vi "evaluation.vi"() -> ()   [LabVIEW 2017]
panel:
  in  "行程测试":bool
  in  "控制板调试":bool
  out "周期稳定性":dbl[](array[numeric])
  out "线性传感器基本误差":dbl[](array[numeric])
  out "重复性误差 R":dbl[](array[numeric])
  out "线性误差":dbl[](array[numeric])
  out "压力传感器系统误差 LH":dbl[](array[numeric])
  out "满量程输出yfs V":dbl[](array[numeric])
  out "温漂":dbl[](array[numeric])
  out "迟滞":dbl[](array[numeric])
  in  "计算参数":bool
  in  "退出":bool
  out "常温索引":i32
  out "XY图":cluster{dbl[], dbl[]}(graph)
  out "显示曲线界面":cluster{dbl[], dbl[]}[][](array[cluster])
  in  "传感器曲线图显示":T1(ring)
  in  "压力下限kPa":dbl
  in  "压力上限kPa":dbl=15000.0
  out "时漂":dbl[](array[numeric])
  out "曲线信息":string[][](array[string])
  in  "压力点个数":i32=6
  in  "检定次数":i32=3
  in  "行程采集文件名":string="202293_1902_700"
  in  "时漂文件名":string="2022917_1702_20.0"
  # "多通道 传感器评估系统"
  # "1"
  # "2"
  # "3"
  # "4"
  # "5"
  # "6"
  # "7"
  # "8"
  # "9"
  # "10"
  # "注意：\n请在计算参数前，先进行行程测试。\n选择传感器索引，获取相关传感器曲线图。"
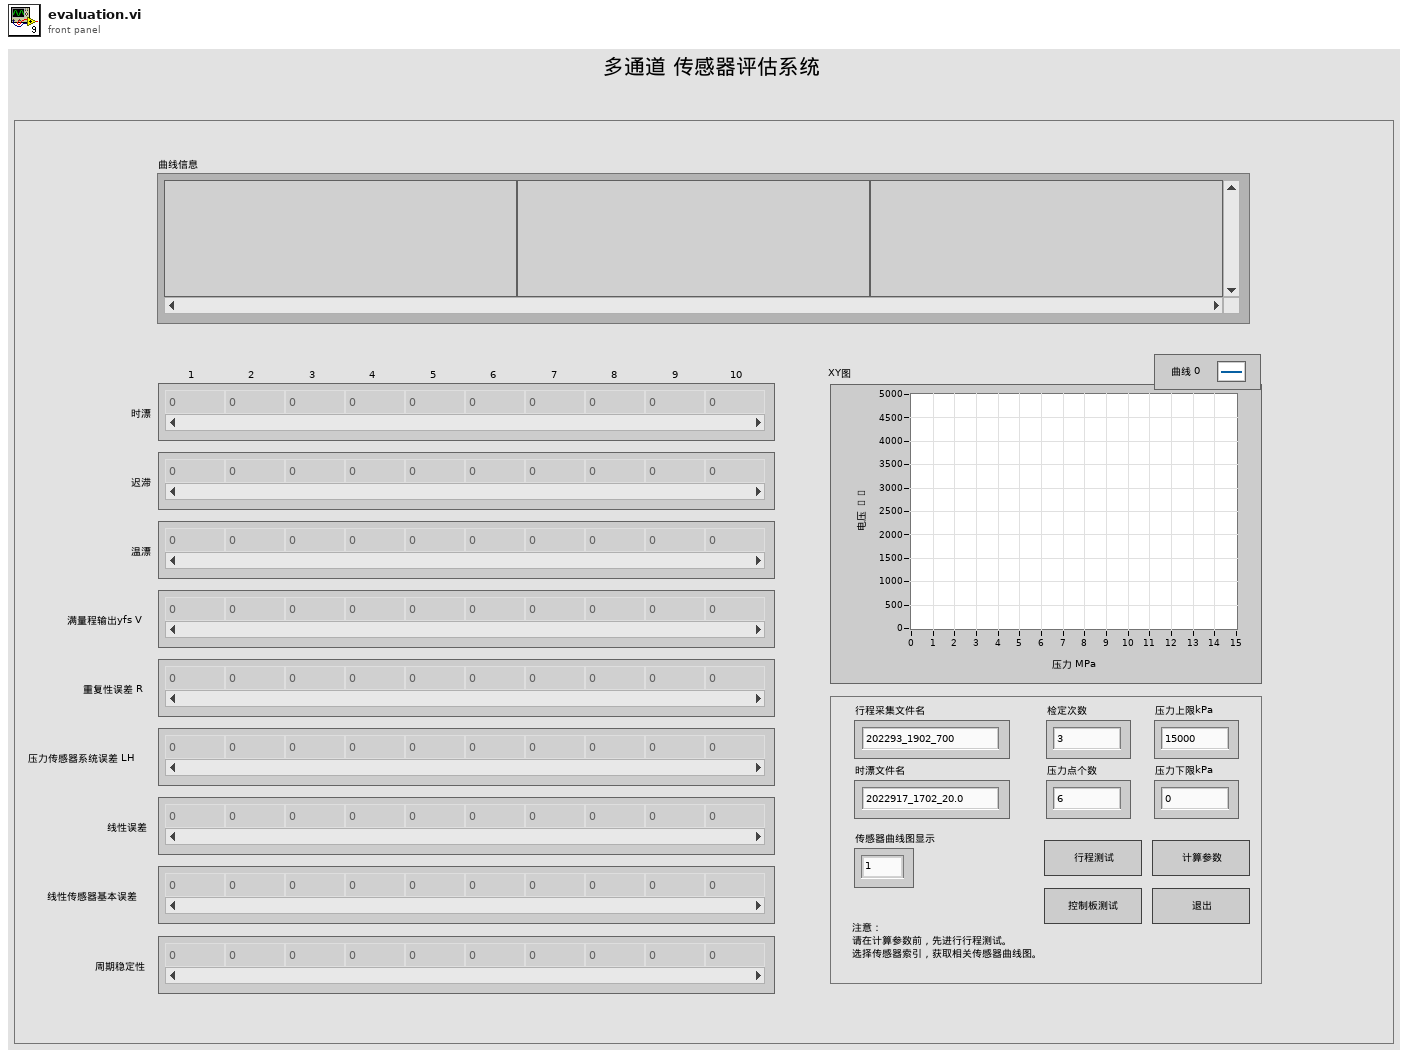
[diagram p1: front panel]
types:
  T1 = enum16{"1", "2", "3", "4", "5", "6", "7", "8", "9", "10"}
  T2 = enum32{"Invalid", "Standard", "Closed", "Hidden", "Minimized", "Maximized"}
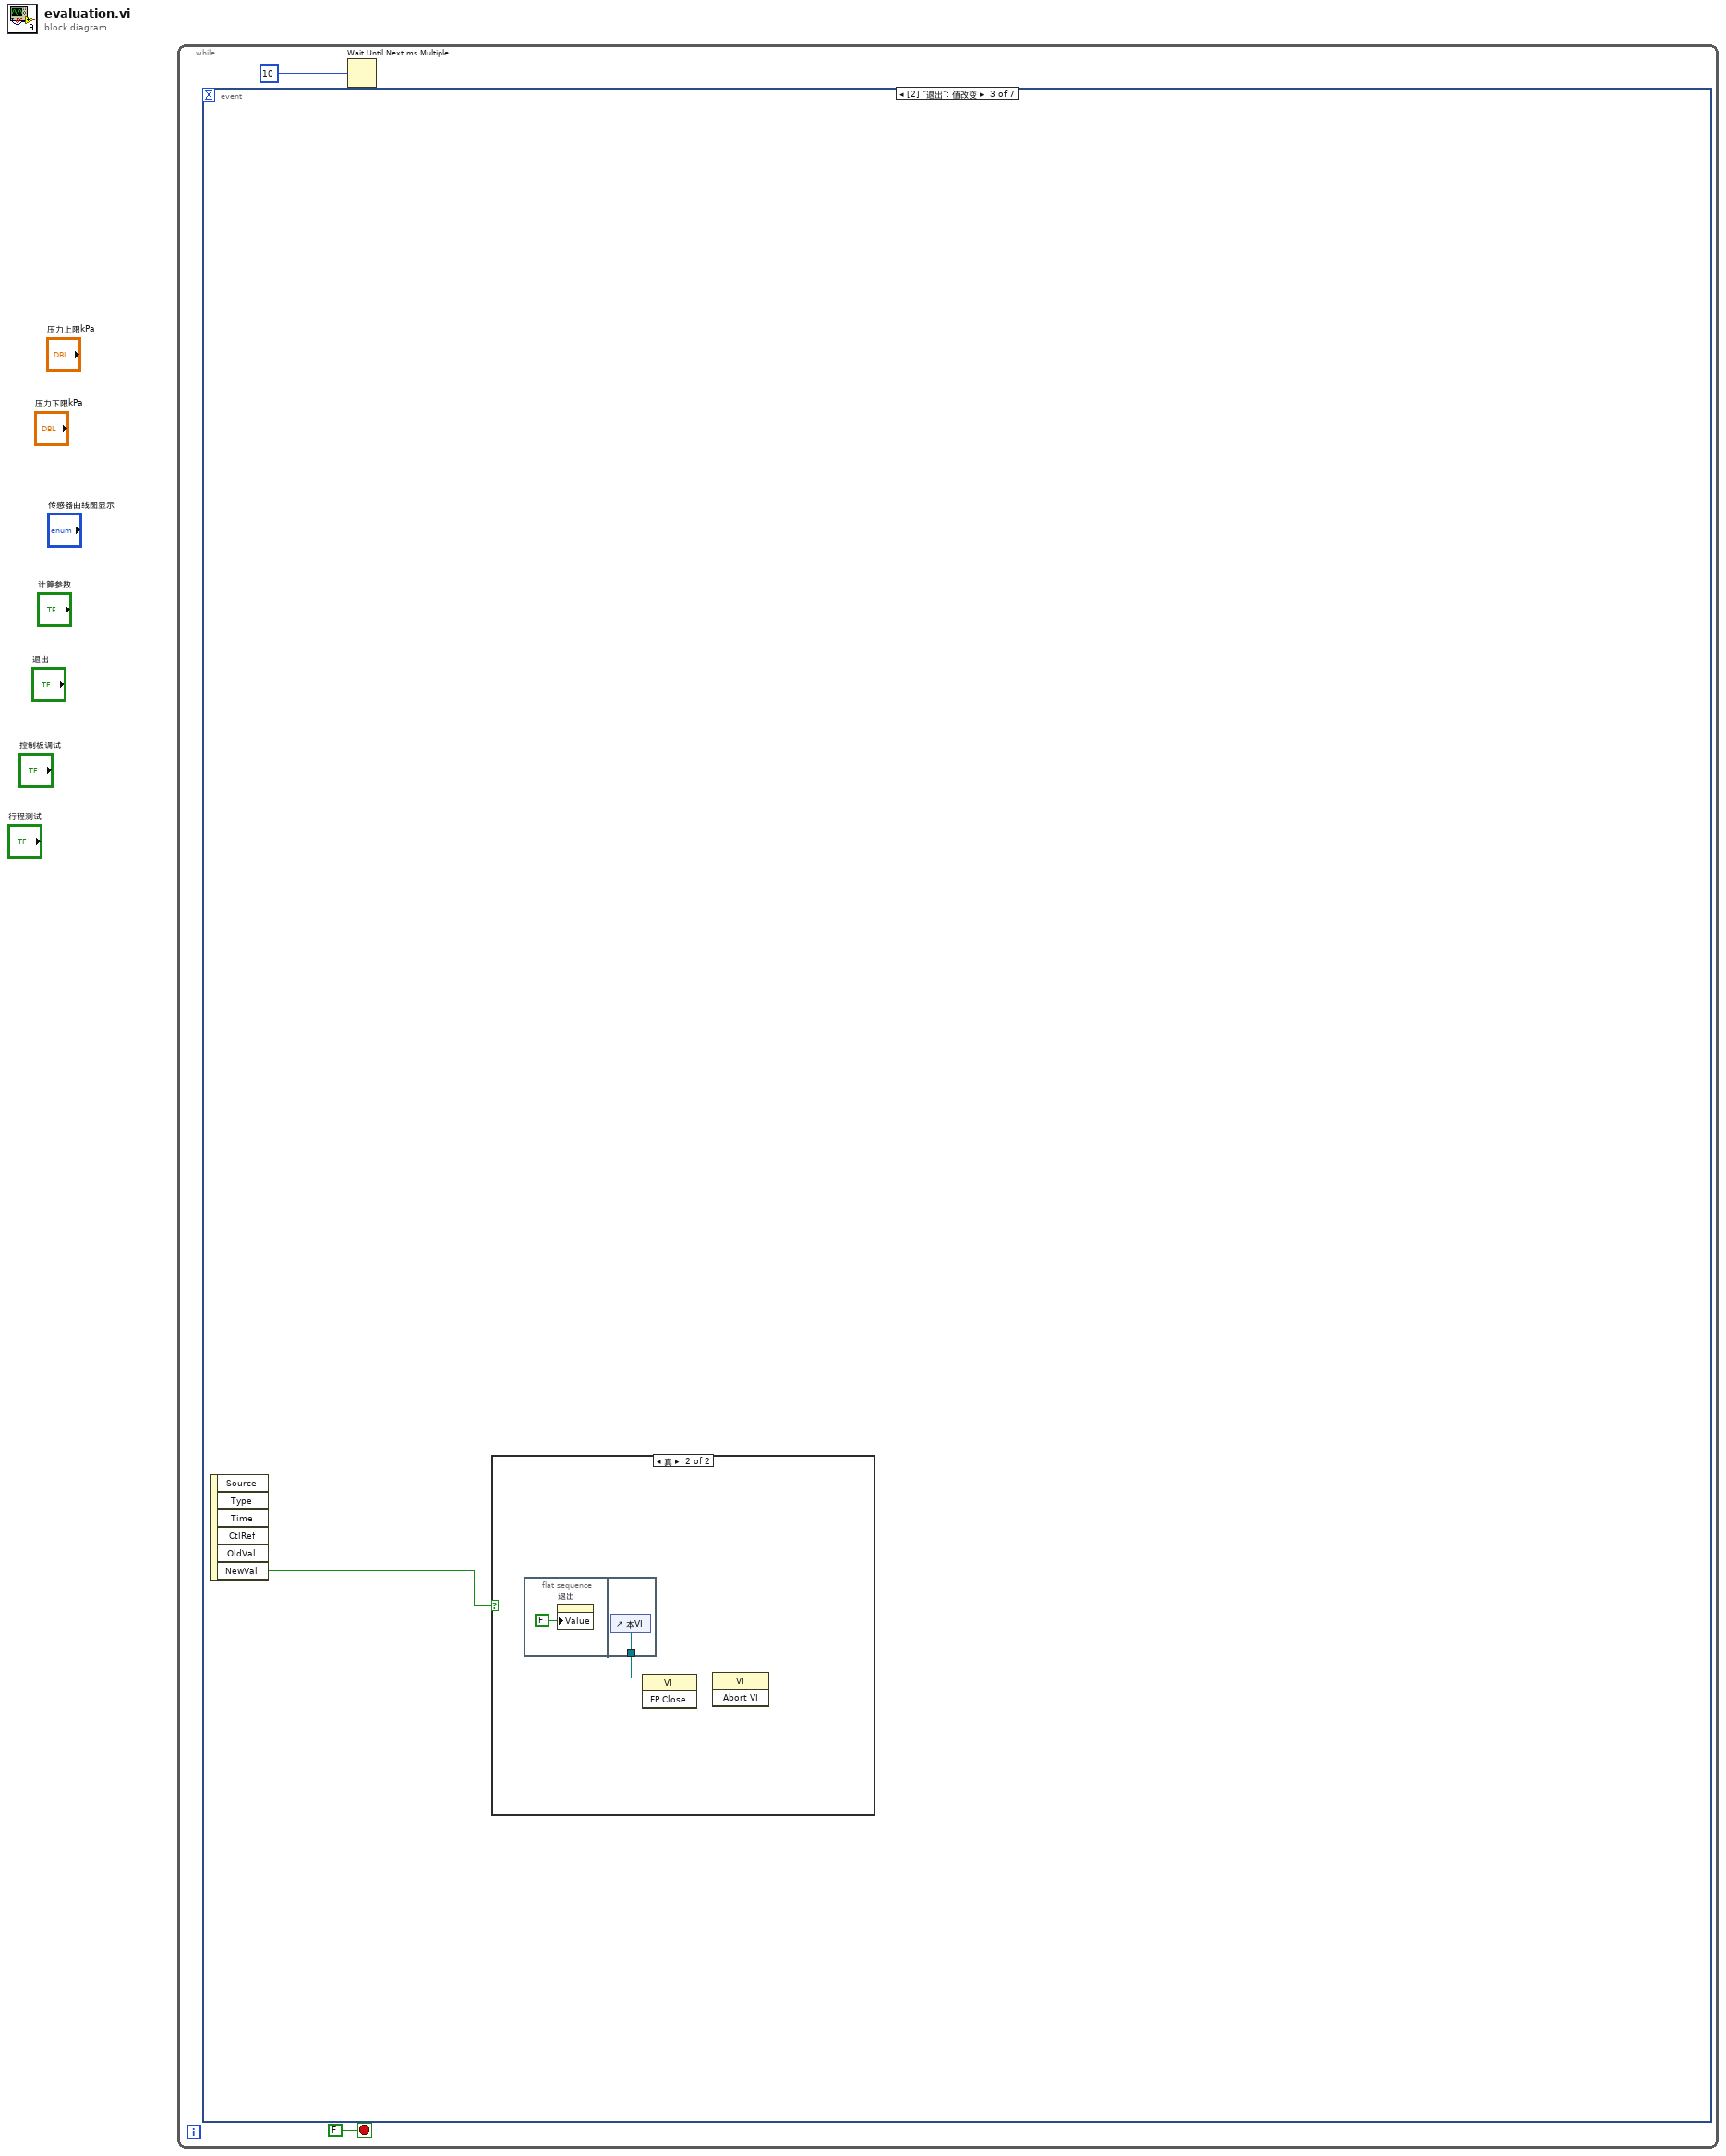
[diagram p0: block diagram]
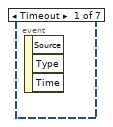
[diagram p2: hidden frame]
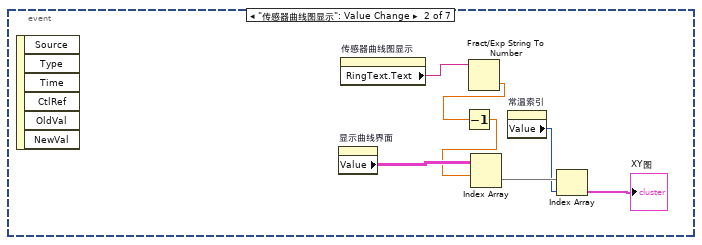
[diagram p3: hidden frame]
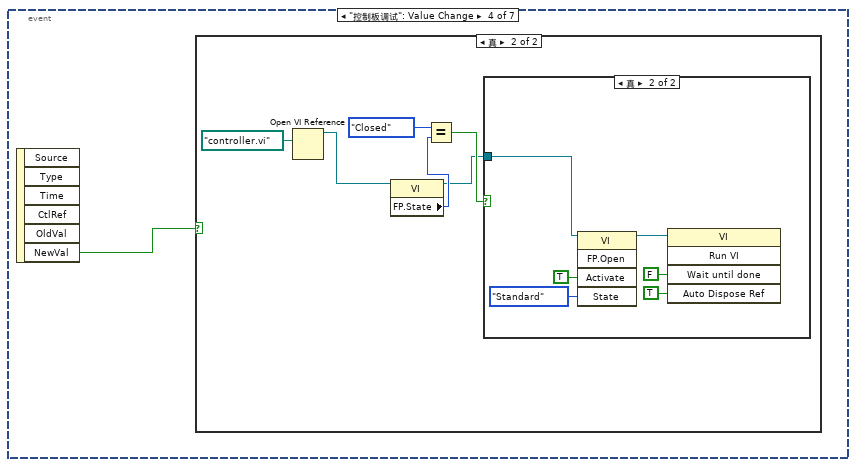
[diagram p5: hidden frame]
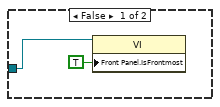
[diagram p7: hidden frame]
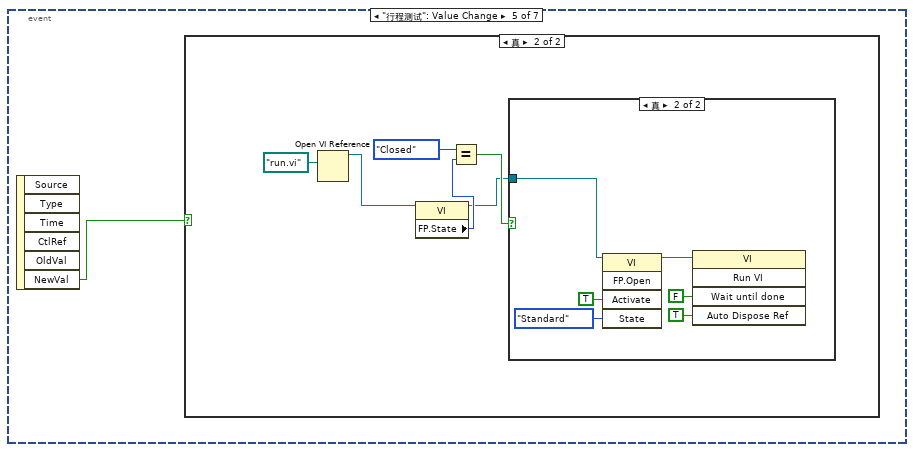
[diagram p8: hidden frame]
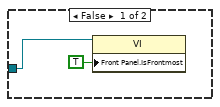
[diagram p10: hidden frame]
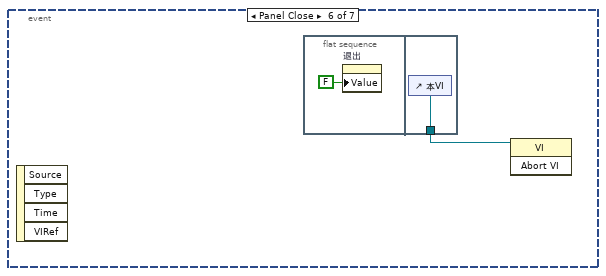
[diagram p11: hidden frame]
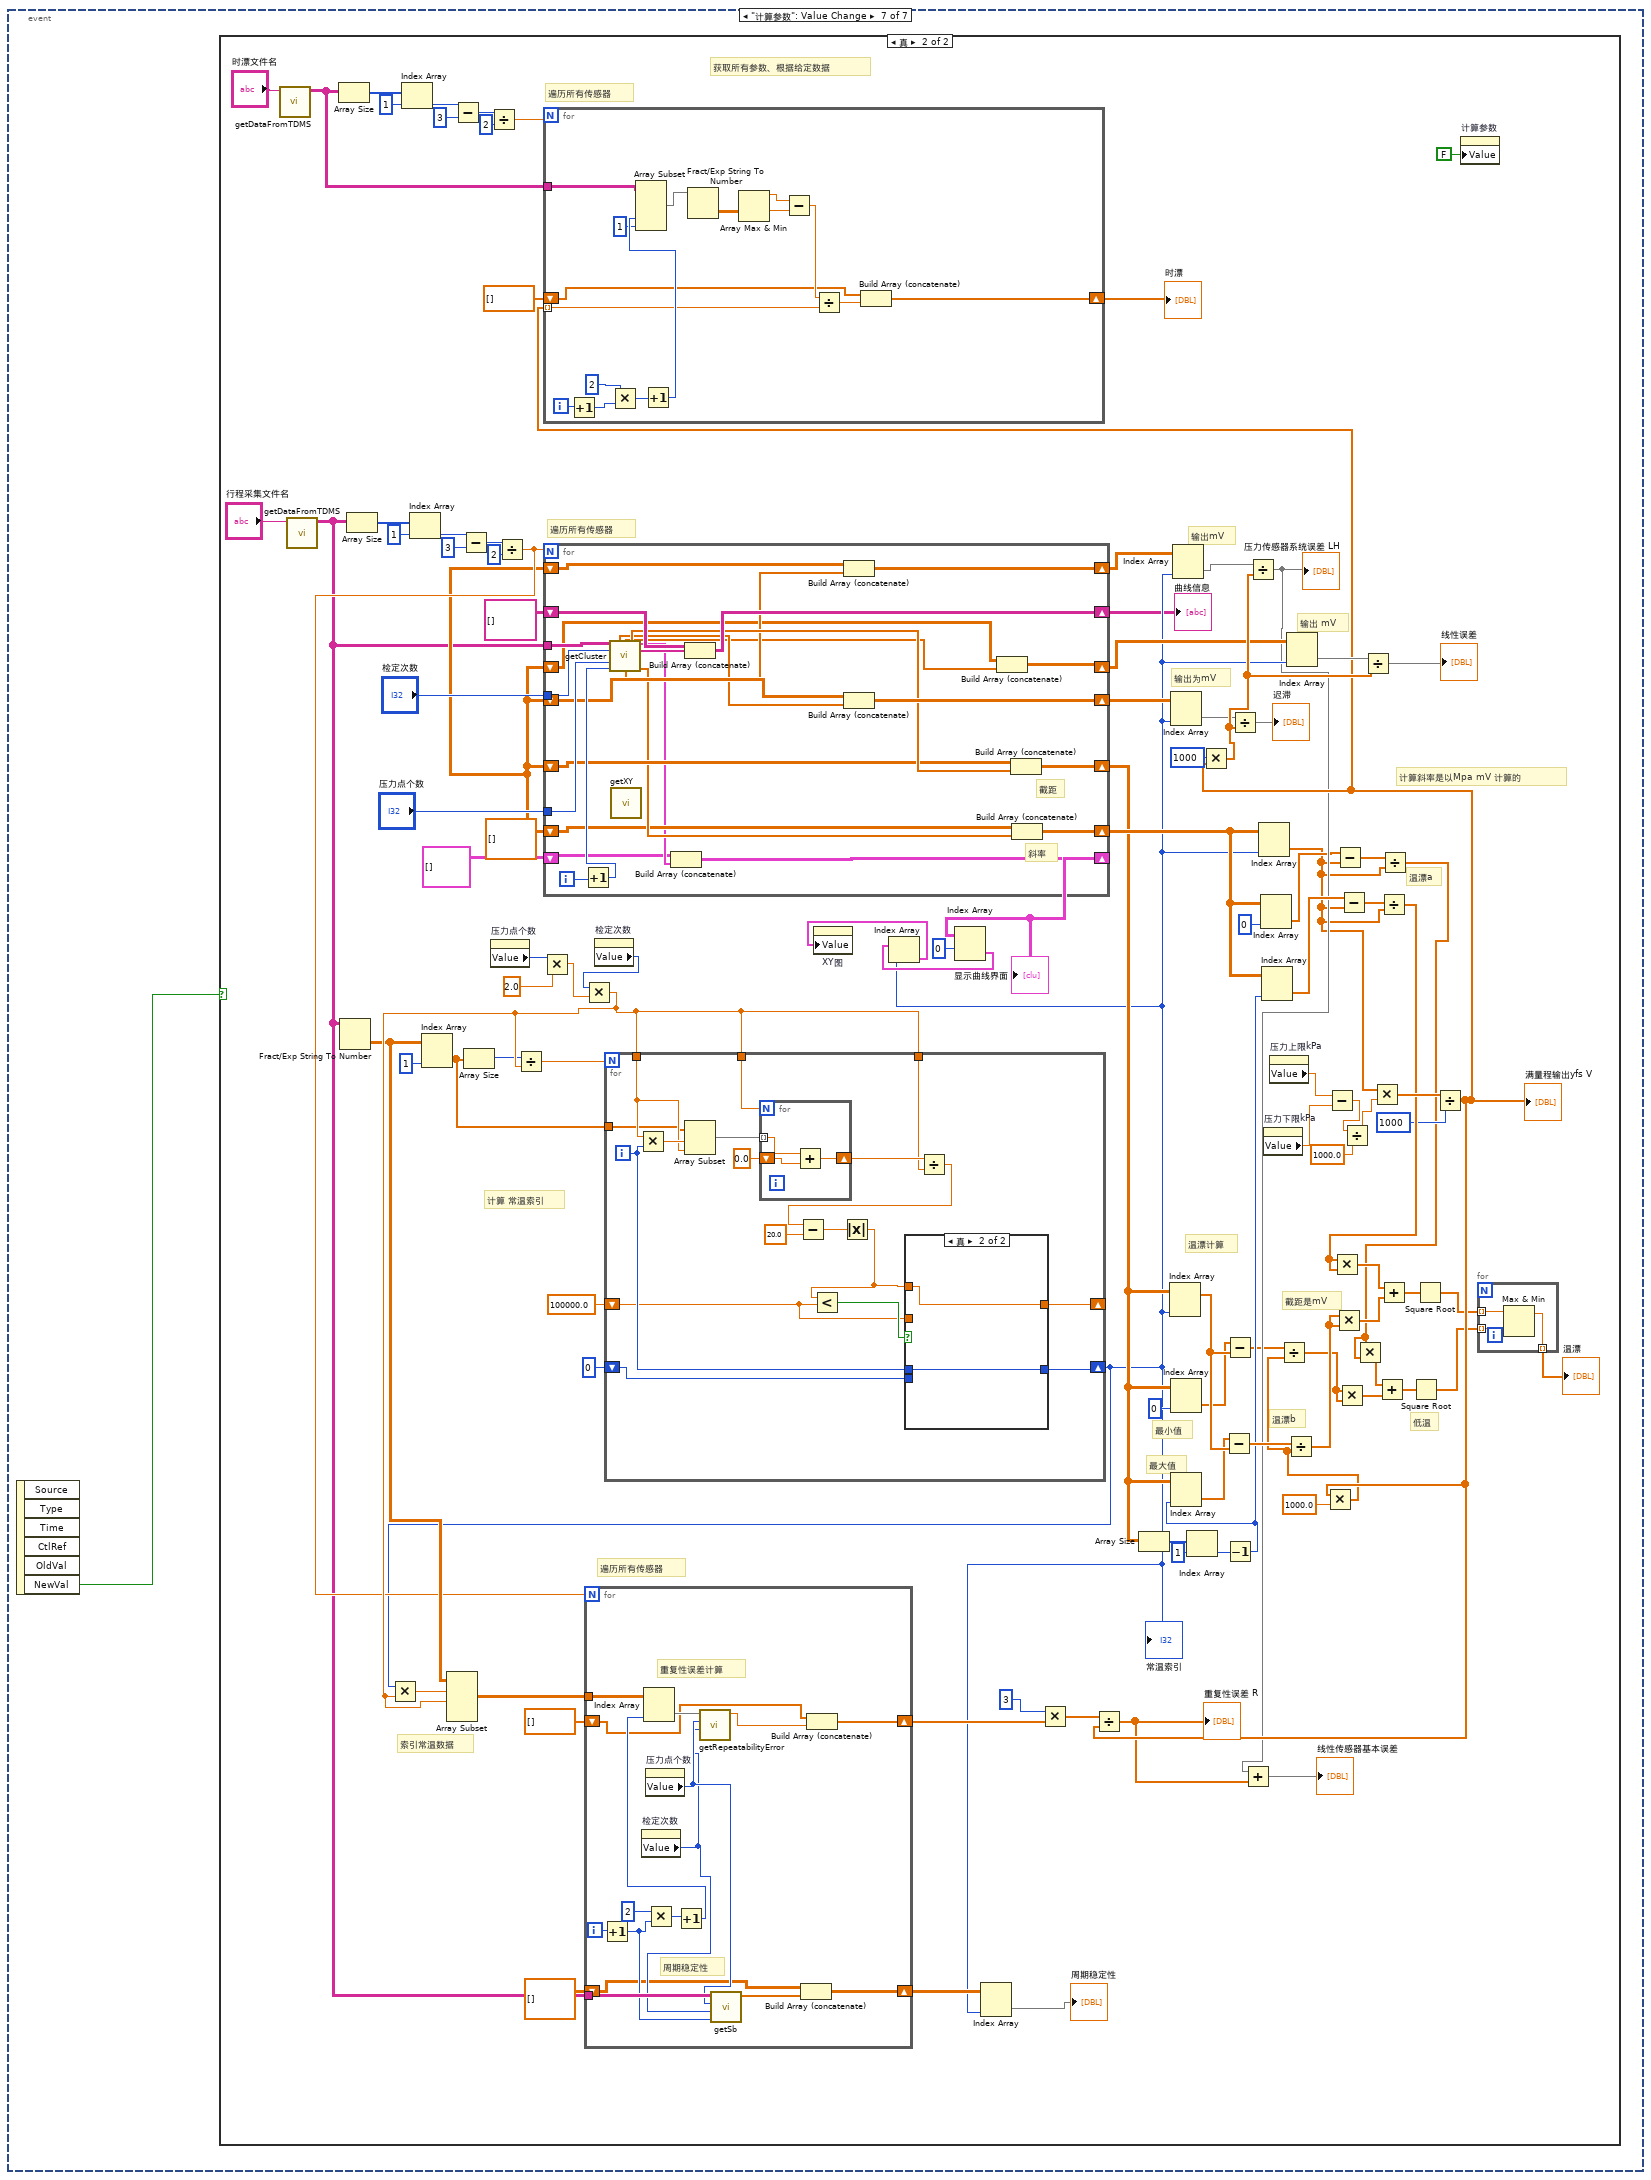
[diagram p12: hidden frame]
diagram:
  n1 = while {
    stop <- FALSE stop-if-true
    n2 = event shown="[2] \"退出\": 值改变" {
      selector: _ -> [_ _ _ _ _ _ _]
      dyn-events: _ -> [_ _ _ _ _ _ _]
      timeout: _ -> [_ _ _ _ _ _ _]
      event Timeout {
        n3 = event-data() -> ()  [unwired: 1 in, 3 out]
      }
      event "传感器曲线图显示": Value Change {
        n4 = event-data() -> ()  [unwired: 1 in, 6 out]
        n5 = property on="显示曲线界面" class="Arr (严格)"() -> ("Value"=w8:cluster{dbl[], dbl[]}[][])  [unwired: 2 in, 2 out]
        n6 = property on="传感器曲线图显示" class="Enum (严格)"() -> ("RingText.Text"=w9:string)  [unwired: 2 in, 2 out]
        n7 = Fract/Exp String To Number(string=w9) -> (number=w4:dbl)  [unwired: 3 in, 1 out]
        n8 = Decrement(x=w4) -> (x-1=w3:dbl)
        n9 = Index Array(array=w8, index (row)=w3) -> (element=w7:cluster{dbl[], dbl[]}[])  [unwired: 1 in]
        n10 = property on="常温索引" class="DigNum (严格)"() -> ("Value"=w6:i32)  [unwired: 2 in, 2 out]
        n11 = Index Array(array=w7, index=w6) -> (element=→"XY图":cluster{dbl[], dbl[]})
      }
      event "退出": Value Change {
        n12 = event-data() -> ("NewVal"=w10:bool)  [unwired: 1 in, 5 out]
        n13 = case shown="真" w10 {
          frame False {
          }
          frame True {
            n14 = flat-sequence {
              tunnel: [w14] -> w12
              frame #0 {
                n15 = property on="退出" class="Bool (严格)"("Value"=FALSE ("退出")) -> ()  [unwired: 2 in, 2 out]
              }
              frame #1 {
                n16 = control-ref of="本VI"() -> (w14:refnum<vi>)
              }
            }
            n17 = invoke class="VI" method="FP.Close"(reference=w12) -> (reference out=w11:refnum<vi>)  [unwired: 2 in, 2 out]
            n18 = invoke class="VI" method="Abort VI"(reference=w11) -> ()  [unwired: 2 in, 3 out]
          }
        }
      }
      event "控制板调试": Value Change {
        n19 = event-data() -> ("NewVal"=w15:bool)  [unwired: 1 in, 5 out]
        n20 = case shown="真" w15 {
          frame False {
          }
          frame True {
            n21 = Open VI Reference(vi path=path "controller.vi" ("VI路径")) -> (vi reference=w16:refnum<vi>)  [unwired: 5 in, 1 out]
            n22 = property class="VI"(reference=w16) -> (reference out=w17:refnum<vi>, "FP.State"=w20:T2)  [unwired: 1 in, 1 out]
            n23 = Equal?(x=T2."Closed", y=w20) -> (x = y?=w18:bool)
            n24 = case shown="真" w18 {
              tunnel: w17 -> [w22 w24]
              frame False {
                n25 = property class="VI"(reference=w22, "Front Panel.IsFrontmost"=TRUE ("前面板窗口:在最前")) -> ()  [unwired: 1 in, 2 out]
              }
              frame True {
                n26 = invoke class="VI" method="FP.Open"(reference=w24, "Activate"=TRUE ("激活？"), "State"=T2."Standard" ("状态")) -> (reference out=w27:refnum<vi>)  [unwired: 2 in, 4 out]
                n27 = invoke class="VI" method="Run VI"(reference=w27, "Wait until done"=FALSE ("结束前等待"), "Auto Dispose Ref"=TRUE ("自动销毁引用")) -> ()  [unwired: 2 in, 5 out]
              }
            }
          }
        }
      }
      event "行程测试": Value Change {
        n28 = event-data() -> ("NewVal"=w30:bool)  [unwired: 1 in, 5 out]
        n29 = case shown="真" w30 {
          frame False {
          }
          frame True {
            n30 = Open VI Reference(vi path=path "run.vi" ("VI路径")) -> (vi reference=w31:refnum<vi>)  [unwired: 5 in, 1 out]
            n31 = property class="VI"(reference=w31) -> (reference out=w32:refnum<vi>, "FP.State"=w35:T2)  [unwired: 1 in, 1 out]
            n32 = Equal?(x=T2."Closed", y=w35) -> (x = y?=w33:bool)
            n33 = case shown="真" w33 {
              tunnel: w32 -> [w37 w39]
              frame False {
                n34 = property class="VI"(reference=w37, "Front Panel.IsFrontmost"=TRUE ("前面板窗口:在最前")) -> ()  [unwired: 1 in, 2 out]
              }
              frame True {
                n35 = invoke class="VI" method="FP.Open"(reference=w39, "Activate"=TRUE ("激活？"), "State"=T2."Standard" ("状态")) -> (reference out=w42:refnum<vi>)  [unwired: 2 in, 4 out]
                n36 = invoke class="VI" method="Run VI"(reference=w42, "Wait until done"=FALSE ("结束前等待"), "Auto Dispose Ref"=TRUE ("自动销毁引用")) -> ()  [unwired: 2 in, 5 out]
              }
            }
          }
        }
      }
      event Panel Close {
        n37 = event-data() -> ()  [unwired: 1 in, 4 out]
        n38 = flat-sequence {
          tunnel: [w47] -> w45
          frame #0 {
            n39 = property on="退出" class="Bool (严格)"("Value"=FALSE ("退出")) -> ()  [unwired: 2 in, 2 out]
          }
          frame #1 {
            n40 = control-ref of="本VI"() -> (w47:refnum<vi>)
          }
        }
        n41 = invoke class="VI" method="Abort VI"(reference=w45) -> ()  [unwired: 2 in, 3 out]
      }
      event "计算参数": Value Change {
        n42 = event-data() -> ("NewVal"=w48:bool)  [unwired: 1 in, 5 out]
        n43 = case shown="真" w48 {
          frame False {
          }
          frame True {
            w83 = dbl[][] []
            # "低温"
            # "索引常温数据"
            # "输出 mV"
            # "输出mV"
            # "遍历所有传感器"
            # "输出为mV"
            # "截距是mV"
            # "计算斜率是以Mpa mV 计算的"
            # "温漂b"
            # "温漂a"
            # "最大值"
            # "最小值"
            # "计算 常温索引"
            # "温漂计算"
            # "遍历所有传感器"
            # "遍历所有传感器"
            # "获取所有参数、根据给定数据"
            n44 = call "getDataFromTDMS.vi"("文件名称"="时漂文件名") -> ("数据"=w112:string[][])  [unwired: 10 in]
            n45 = call "getDataFromTDMS.vi"("文件名称"="行程采集文件名") -> ("数据"=w77:string[][])  [unwired: 10 in]
            n46 = Array Size(array=w112) -> (size(s)=w108:i32[])
            n47 = Fract/Exp String To Number(string=w77) -> (number=w142:dbl[][])  [unwired: 3 in, 1 out]
            n48 = Array Size(array=w77) -> (size(s)=w101:i32[])
            n49 = Index Array(array=w108, index=1 ("索引")) -> (element=w109:i32)
            n50 = Index Array(array=w101, index=1 ("索引")) -> (element=w102:i32)
            n51 = Index Array(array=w142, index (col)=1 ("禁用的索引 (列)")) -> (element=w119:dbl[])  [unwired: 1 in]
            n52 = Subtract(x=w109, y=3) -> (x-y=w110:i32)
            n53 = Subtract(x=w102, y=3) -> (x-y=w103:i32)
            n54 = Array Size(array=w119) -> (size(s)=w117:i32)
            n55 = Divide(x=w110, y=2) -> (x/y=w111:dbl)
            n56 = property on="压力点个数" class="DigNum (严格)"() -> ("Value"=w114:i32)  [unwired: 2 in, 2 out]
            n57 = Divide(x=w103, y=2) -> (x/y=w141:dbl)
            n58 = Multiply(x=w114, y=2.0) -> (x*y=w115:dbl)
            n59 = for {
              N: w141 -> [_]
              tunnel: w77 -> [w240]
              tunnel: "检定次数" -> [w239]
              tunnel: "压力点个数" -> [w238]
              shift-right: [w234] -> w72
              shift-left: string[][] [] -> [w236]
              shift-right: [w233] -> w120
              shift-left: w83 -> [w232]
              shift-right: [w229] -> w121
              shift-left: w83 -> [w230]
              shift-right: [w227] -> w124
              shift-left: w83 -> [w226]
              shift-right: [w223] -> w148
              shift-left: w83 -> [w222]
              shift-right: [w220] -> w150
              shift-left: cluster{dbl[], dbl[]}[][] [] -> [w219]
              shift-right: [w216] -> w153
              shift-left: w83 -> [w217]
              i -> [w241]
              # "截距"
              # "斜率"
              n60 = Increment(x=w241) -> (x+1=w237:i32)
              n61 = call "getCluster.vi"("数据"=w240, "检定次数"=w239, "压力点个数"=w238, "传感器索引（1开始）"=w237) -> ("迟滞mV"=w225:dbl[], "线性误差"=w218:dbl[], "截距数组"=w231:dbl[], "结果簇"=w221:cluster{dbl[], dbl[]}[], "曲线信息"=w235:string[], "系统误差mV"=w224:dbl[], "斜率数组"=w228:dbl[])  [unwired: 4 in, 1 out]
              n62 = call "getXY.vi"() -> ()  [unwired: 8 in, 8 out]
              n63 = Build Array (concatenate)(w219, w221) -> (w220:cluster{dbl[], dbl[]}[][])
              n64 = Build Array (concatenate)(w236, w235) -> (w234:string[][])
              n65 = Build Array (concatenate)(w222, w224) -> (w223:dbl[][])
              n66 = Build Array (concatenate)(w232, w225) -> (w233:dbl[][])
              n67 = Build Array (concatenate)(w217, w218) -> (w216:dbl[][])
              n68 = Build Array (concatenate)(w230, w231) -> (w229:dbl[][])
              n69 = Build Array (concatenate)(w226, w228) -> (w227:dbl[][])
            }
            "曲线信息" <- w72
            "显示曲线界面" <- w150
            n70 = property on="检定次数" class="DigNum (严格)"() -> ("Value"=w116:i32)  [unwired: 2 in, 2 out]
            n71 = Multiply(x=w116, y=w115) -> (x*y=w144:dbl)
            n72 = Divide(x=w117, y=w144) -> (x/y=w118:dbl)
            n73 = for {
              N: w118 -> [_]
              tunnel: w144 -> [w191]
              tunnel: w144 -> [w190]
              tunnel: w119 -> [w188]
              tunnel: w144 -> [w186]
              shift-right: [w177] -> _
              shift-left: 100000.0 -> [w176]
              shift-right: [w181] -> w73
              shift-left: 0 -> [w180]
              i -> [w182]
              n74 = Multiply(x=w191, y=w182) -> (x*y=w192:dbl)
              n75 = Array Subset(array=w188, index=w192, length=w191) -> (w189:dbl[])
              n76 = for {
                N: w190 -> [_]
                tunnel: w189 -> [w199] mode=indexing
                shift-right: [w198] -> w187
                shift-left: 0.0 -> [w197]
                n77 = Add(x=w199, y=w197) -> (x+y=w198:dbl)
              }
              n78 = Divide(x=w187, y=w186) -> (x/y=w185:dbl)
              n79 = Subtract(x=w185, y=20.0) -> (x-y=w183:dbl)
              n80 = Absolute Value(x=w183) -> (abs(x)=w178:dbl)
              n81 = Less?(x=w178, y=w176) -> (x < y?=w179:bool)
              n82 = case shown="真" w179 {
                tunnel: w182 -> [_ w196]
                tunnel: [w194 w196] -> w181
                tunnel: w180 -> [w194 _]
                tunnel: w178 -> [_ w195]
                tunnel: [w193 w195] -> w177
                tunnel: w176 -> [w193 _]
                frame False {
                }
                frame True {
                }
              }
            }
            "常温索引" <- w73
            n83 = Multiply(x=w73, y=w144) -> (x*y=w143:dbl)
            n84 = Array Subset(array=w142, index (row)=w143, length (row)=w144) -> (w145:dbl[][])  [unwired: 2 in]
            n85 = for {
              N: w141 -> [_]
              tunnel: w145 -> [w171]
              shift-right: [w167] -> w146
              shift-left: dbl[] [] -> [w166]
              tunnel: w77 -> [w165]
              shift-right: [w160] -> w74
              shift-left: dbl[][] [] -> [w159]
              i -> [w173]
              # "周期稳定性"
              # "重复性误差计算"
              n86 = Increment(x=w173) -> (x+1=w162:i32)
              n87 = property on="检定次数" class="DigNum (严格)"() -> ("Value"=w163:i32)  [unwired: 2 in, 2 out]
              n88 = property on="压力点个数" class="DigNum (严格)"() -> ("Value"=w164:i32)  [unwired: 2 in, 2 out]
              n89 = Multiply(x=2, y=w162) -> (x*y=w172:i32)
              n90 = Increment(x=w172) -> (x+1=w170:i32)
              n91 = Index Array(array=w171, index (col)=w170) -> (element=w169:dbl[])  [unwired: 1 in]
              n92 = call "getRepeatabilityError.vi"("检定次数"=w163, "压力点个数"=w164, "温度点一维数组数据"=w169) -> ("标准偏差"=w168:dbl)  [unwired: 8 in]
              n93 = call "getSb.vi"("传感器索引"=w162, "检定次数"=w163, "压力点个数"=w164, "数据"=w165) -> ("周期稳定性"=w161:dbl[])  [unwired: 7 in]
              n94 = Build Array (concatenate)(w159, w161) -> (w160:dbl[][])
              n95 = Build Array (concatenate)(w166, w168) -> (w167:dbl[])
            }
            n96 = Index Array(array=w150, index (row)=0 ("索引 (行)")) -> (element=w151:cluster{dbl[], dbl[]}[])  [unwired: 1 in]
            n97 = Index Array(array=w151, index=w73) -> (element=w152:cluster{dbl[], dbl[]})
            n98 = property on="XY图" class="XYGraph (严格)"("Value"=w152) -> ()  [unwired: 2 in, 2 out]
            n99 = Index Array(array=w74, index (col)=w73) -> (element=→"周期稳定性":dbl[])  [unwired: 1 in]
            n100 = Multiply(x=3, y=w146) -> (x*y=w147:dbl[])
            n101 = Array Size(array=w121) -> (size(s)=w122:i32[])
            n102 = Index Array(array=w121, index (col)=w73) -> (element=w136:dbl[])  [unwired: 1 in]
            n103 = Index Array(array=w120, index (col)=w73) -> (element=w140:dbl[])  [unwired: 1 in]
            n104 = Index Array(array=w121, index (col)=0 ("禁用的索引 (列)")) -> (element=w129:dbl[])  [unwired: 1 in]
            n105 = Index Array(array=w148, index (col)=w73) -> (element=w149:dbl[])  [unwired: 1 in]
            n106 = Index Array(array=w122, index=1 ("索引")) -> (element=w123:i32)
            n107 = Subtract(x=w129, y=w136) -> (x-y=w61:dbl[])
            n108 = Decrement(x=w123) -> (x-1=w125:i32)
            n109 = Index Array(array=w121, index (col)=w125) -> (element=w130:dbl[])  [unwired: 1 in]
            n110 = Subtract(x=w130, y=w136) -> (x-y=w128:dbl[])
            n111 = Index Array(array=w124, index (col)=w73) -> (element=w53:dbl[])  [unwired: 1 in]
            n112 = Index Array(array=w124, index (col)=0 ("禁用的索引 (列)")) -> (element=w55:dbl[])  [unwired: 1 in]
            n113 = Index Array(array=w124, index (col)=w125) -> (element=w126:dbl[])  [unwired: 1 in]
            n114 = property on="压力下限kPa" class="DigNum (严格)"() -> ("Value"=w138:dbl)  [unwired: 2 in, 2 out]
            n115 = property on="压力上限kPa" class="DigNum (严格)"() -> ("Value"=w137:dbl)  [unwired: 2 in, 2 out]
            n116 = Index Array(array=w153, index (col)=w73) -> (element=w155:dbl[])  [unwired: 1 in]
            n117 = Subtract(x=w137, y=w138) -> (x-y=w64:dbl)
            n118 = Subtract(x=w55, y=w53) -> (x-y=w54:dbl[])
            n119 = Subtract(x=w126, y=w53) -> (x-y=w127:dbl[])
            n120 = Divide(x=w64, y=1000.0) -> (x/y=w62:dbl)
            n121 = Multiply(x=w53, y=w62) -> (x*y=w139:dbl[])
            n122 = Divide(x=w127, y=w53) -> (x/y=w132:dbl[])
            n123 = Multiply(x=w132, y=w132) -> (x*y=w134:dbl[])
            n124 = Divide(x=w54, y=w53) -> (x/y=w52:dbl[])
            n125 = Multiply(x=w52, y=w52) -> (x*y=w56:dbl[])
            n126 = Divide(x=w139, y=1000) -> (x/y=w70:dbl[])
            "满量程输出yfs V" <- w70
            n127 = for {
              N: w111 -> [_]
              tunnel: w112 -> [w215]
              tunnel: w70 -> [w204] mode=indexing
              shift-right: [w202] -> w113
              shift-left: dbl[] [] -> [w201]
              i -> [w214]
              n128 = Increment(x=w214) -> (x+1=w213:i32)
              n129 = Multiply(x=2, y=w213) -> (x*y=w211:i32)
              n130 = Increment(x=w211) -> (x+1=w210:i32)
              n131 = Array Subset(array=w215, index (col)=w210, length (col)=1 ("长度")) -> (w209:string[][])  [unwired: 2 in]
              n132 = Fract/Exp String To Number(string=w209) -> (number=w208:dbl[][])  [unwired: 3 in, 1 out]
              n133 = Array Max & Min(array=w208) -> (max value=w207:dbl, min value=w206:dbl)  [unwired: 2 out]
              n134 = Subtract(x=w207, y=w206) -> (x-y=w205:dbl)
              n135 = Divide(x=w205, y=w204) -> (x/y=w203:dbl)
              n136 = Build Array (concatenate)(w201, w203) -> (w202:dbl[])
            }
            "时漂" <- w113
            n137 = Divide(x=w147, y=w70) -> (x/y=w69:dbl[])
            "重复性误差 R" <- w69
            n138 = Multiply(x=1000, y=w70) -> (x*y=w154:dbl[])
            n139 = Divide(x=w140, y=w154) -> (x/y=→"迟滞":dbl[])
            n140 = Divide(x=w149, y=w154) -> (x/y=w68:dbl[])
            "压力传感器系统误差 LH" <- w68
            n141 = Add(x=w68, y=w69) -> (x+y=→"线性传感器基本误差":dbl[])
            n142 = Multiply(x=w70, y=1000.0) -> (x*y=w60:dbl[])
            n143 = Divide(x=w61, y=w60) -> (x/y=w59:dbl[])
            n144 = Divide(x=w128, y=w60) -> (x/y=w131:dbl[])
            n145 = Multiply(x=w131, y=w131) -> (x*y=w133:dbl[])
            n146 = Multiply(x=w59, y=w59) -> (x*y=w58:dbl[])
            n147 = Divide(x=w155, y=w154) -> (x/y=→"线性误差":dbl[])
            n148 = Add(x=w56, y=w58) -> (x+y=w57:dbl[])
            n149 = Add(x=w134, y=w133) -> (x+y=w135:dbl[])
            n150 = Square Root(x=w57) -> (sqrt(x)=w50:dbl[])
            n151 = Square Root(x=w135) -> (sqrt(x)=w51:dbl[])
            n152 = property on="计算参数" class="Bool (严格)"("Value"=FALSE ("计算参数")) -> ()  [unwired: 2 in, 2 out]
            n153 = for {
              tunnel: w51 -> [w158] mode=indexing
              tunnel: w50 -> [w157] mode=indexing
              tunnel: [w156] -> w49 mode=indexing
              n154 = Max & Min(x=w158, y=w157) -> (max(x,y)=w156:dbl)  [unwired: 1 out]
            }
            "温漂" <- w49
          }
        }
      }
    }
    n155 = Wait Until Next ms Multiple(millisecond multiple=u32 10 ("毫秒倍数")) -> ()  [unwired: 1 out]
  }
